vi "HatchSideCollisionAvoidance.vi"(11 "Intended Hatch Setpoint":dbl) -> (3 "Modified Hatch Setpoint":dbl)   [LabVIEW 2018]
uses:
  Infrastructure/Constants.vi
  Robot Global Data.vi
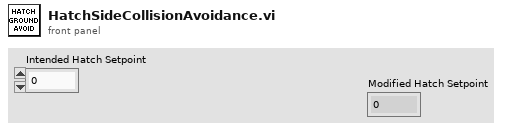
[diagram p1: front panel]
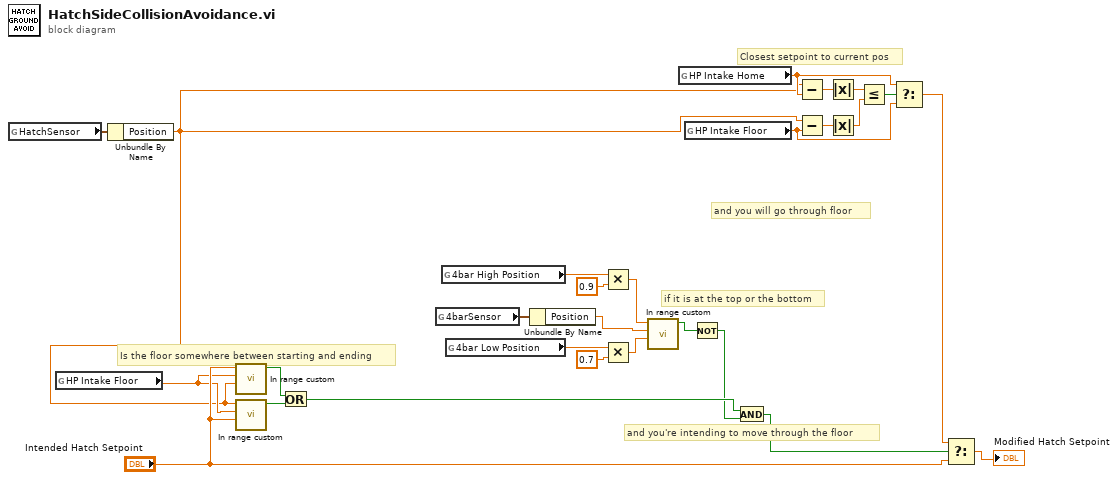
[diagram p0: block diagram]
diagram:
  # "and you're intending to move through the floor"
  # "if it is at the top or the bottom"
  # "and you will go through floor"
  # "Closest setpoint to current pos"
  # "Is the floor somewhere between starting and ending"
  n1 = global read "Robot Global Data.vi" "HatchSensor"() -> (w27:cluster{"Position":dbl, "Velocity":dbl})
  n2 = global read "Constants.vi" "HP Intake Floor"() -> (w6:dbl)
  n3 = Unbundle By Name(w27) -> ("Position"=w5:dbl)
  n4 = call "In range custom.vi"("Lower limit"=w5, "x"=w6, "Upper limit"="Intended Hatch Setpoint") -> ("In range?"=w8:bool)  [unwired: 8 in]
  n5 = call "In range custom.vi"("Lower limit"="Intended Hatch Setpoint", "x"=w6, "Upper limit"=w5) -> ("In range?"=w9:bool)  [unwired: 8 in]
  n6 = Or(x=w8, y=w9) -> (x .or. y?=w13:bool)
  n7 = global read "Robot Global Data.vi" "4barSensor"() -> (w26:cluster{"Position":dbl, "Velocity":dbl})
  n8 = global read "Constants.vi" "4bar High Position"() -> (w16:dbl)
  n9 = global read "Constants.vi" "4bar Low Position"() -> (w25:dbl)
  n10 = Unbundle By Name(w26) -> ("Position"=w2:dbl)
  n11 = Multiply(x=w16, y=0.9) -> (x*y=w3:dbl)
  n12 = Multiply(x=w25, y=0.7) -> (x*y=w1:dbl)
  n13 = call "In range custom.vi"("Lower limit"=w1, "x"=w2, "Upper limit"=w3) -> ("In range?"=w4:bool)  [unwired: 8 in]
  n14 = global read "Constants.vi" "HP Intake Home"() -> (w23:dbl)
  n15 = global read "Constants.vi" "HP Intake Floor"() -> (w22:dbl)
  n16 = Not(x=w4) -> (.not. x?=w10:bool)
  n17 = And(x=w13, y=w10) -> (x .and. y?=w12:bool)
  n18 = Subtract(x=w5, y=w23) -> (x-y=w17:dbl)
  n19 = Subtract(x=w5, y=w22) -> (x-y=w18:dbl)
  n20 = Absolute Value(x=w17) -> (abs(x)=w19:dbl)
  n21 = Absolute Value(x=w18) -> (abs(x)=w20:dbl)
  n22 = Less Or Equal?(x=w19, y=w20) -> (x <= y?=w21:bool)
  n23 = Select(t=w23, s=w21, f=w22) -> (s? t:f=w14:dbl)
  n24 = Select(t=w14, s=w12, f="Intended Hatch Setpoint") -> (s? t:f=→"Modified Hatch Setpoint":dbl)
